vi "SA40144C.20201219 Data Analysis.vi"() -> ()   [LabVIEW 2020]
uses:
  <vilib>/Analysis/baseanly.llb/Mean (DBL).vi
  <userlib>/_OpenG.lib/file/file.llb/Build Path - Traditional__ogtk.vi
  <userlib>/LevyLab/LV to ITX/Data/Data.lvclass
  <userlib>/LevyLab/XY Utilities/xy_utilities.lvlib
  <vilib>/Analysis/NI_AALBase.lvlib
panel:
  in  "Temps to keep (Lifespan)":i32=11
  out "Lifespan vs Temp (hrs)":cluster{i32[], dbl[]}[](graph)
  out "E_a":dbl[](array[numeric])
  out "Arrhenius":T1(graph)
  in  "Temps to keep (Arrhenius fit)":i32=11
  out "G2T vs t":T1(graph)
  out "G4T vs t":T1(graph)
  out "G2T vs t 2D":T1(graph)
  out "G4T vs t  2D":T1(graph)
  in  "Source Voltage":dbl=0.1
  in  "Init Temp":i32=275
  in  "Temp Step":i32=5
  in  "Final Temp":i32=325
  in  "Data File":path=path "G:/My Drive/ansom/Data/PPMS 2/SA40144C.20201219/01 - Temp Sweep/SA40144C.20201219.275K.dat"
  in  "Trimming":i32=400
  in  "Update":bool
  in  "OK":bool
  out "error out":errorcluster
  in  "error in (no error)":errorcluster
  # "2T"
  # "4T"
  # "2T 2D"
  # "4T 2D"
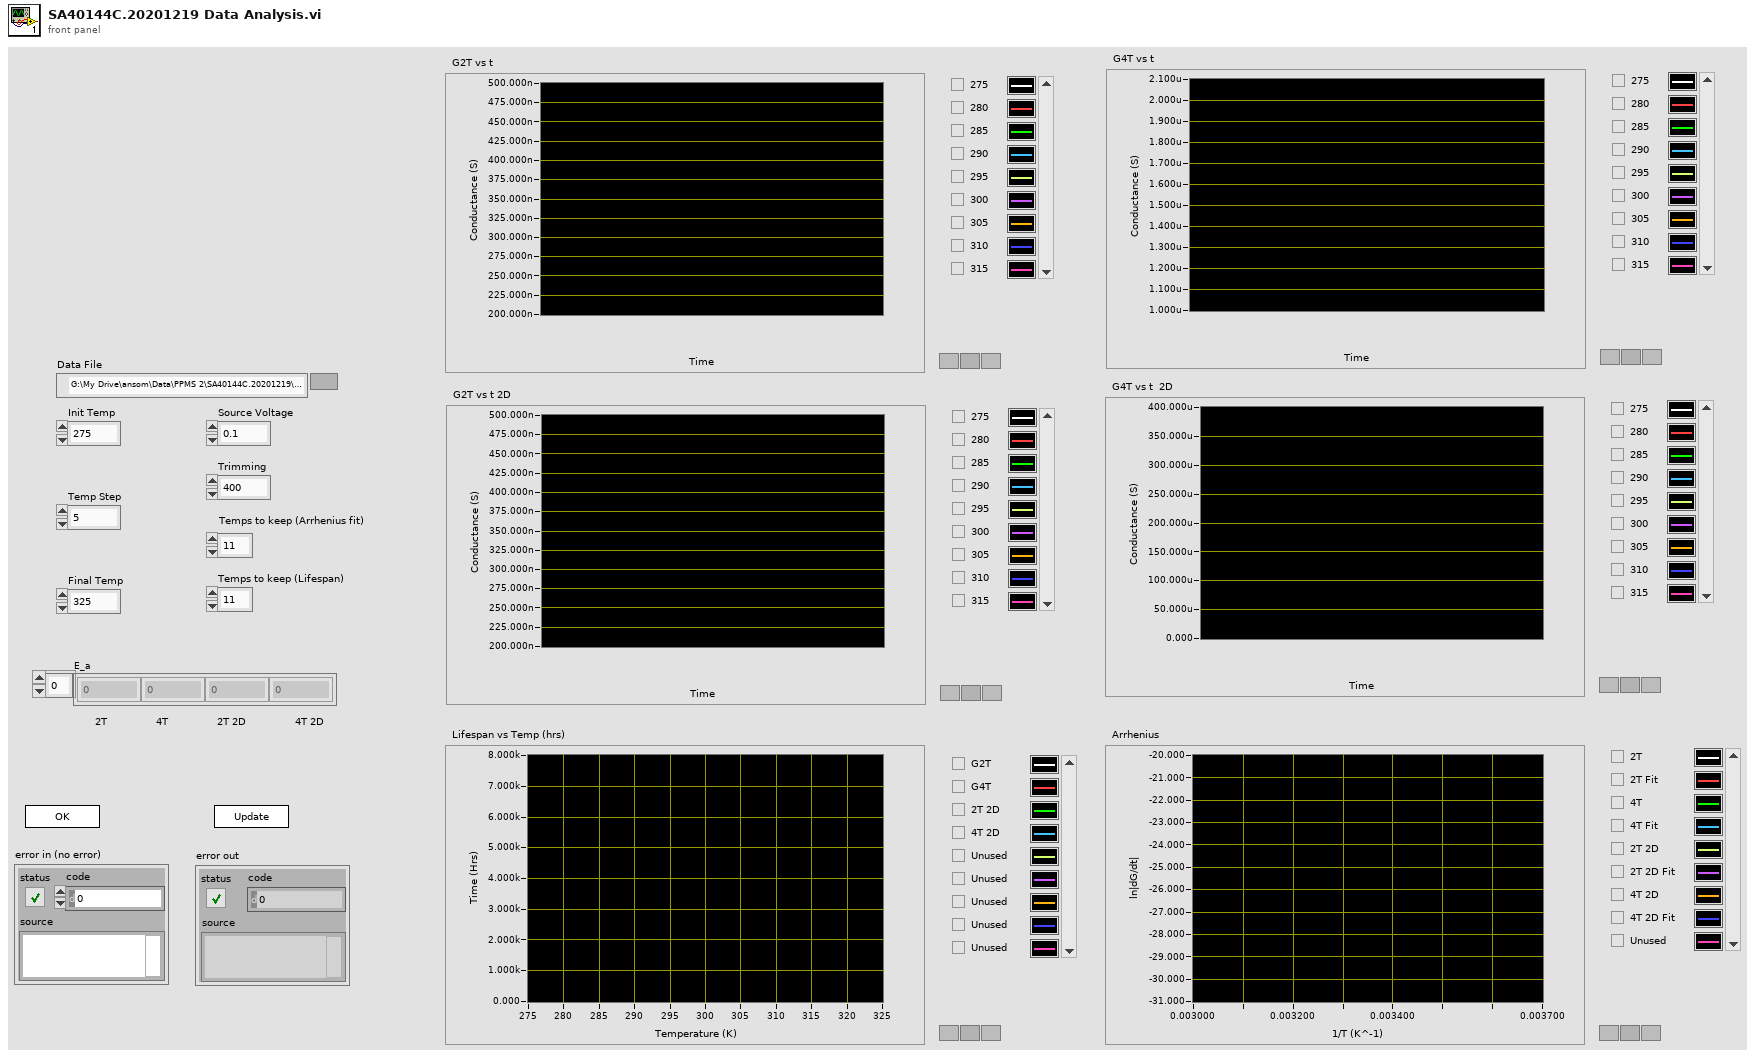
[diagram p1: front panel]
types:
  T1 = cluster{"Data":dbl[], "Best Exponential Fit":dbl[]}[]
  T2 = enum32{"Invalid", "Standard", "Closed", "Hidden", "Minimized", "Maximized"}
  T3 = enum32{"invalid app kind", "Development System", "Run Time System", "Student Edition", "Embedded LabVIEW", "Evaluation", "Custom"}
  T4 = cluster{"Core":cluster{"Current VI Reference":refnum<vi>, "Close Panel on Exit?":bool}, "G2T 1D":cluster{dbl[], dbl[]}[], "G4T 1D":cluster{dbl[], dbl[]}[], "G2T 2D":cluster{dbl[], dbl[]}[], "G4T 2D":cluster{dbl[], dbl[]}[], "Source Voltage":dbl, "Final Temp":i32, "Init Temp":i32, "Temp Step":i32, "Data File":path, "Trimming":i32}
  T5 = cluster{"Current VI Reference":refnum<vi>, "Close Panel on Exit?":bool}
  T6 = typedef "Data.lvclass/Dictionary--cluster.ctl" = cluster{"key":string, "value":variant}
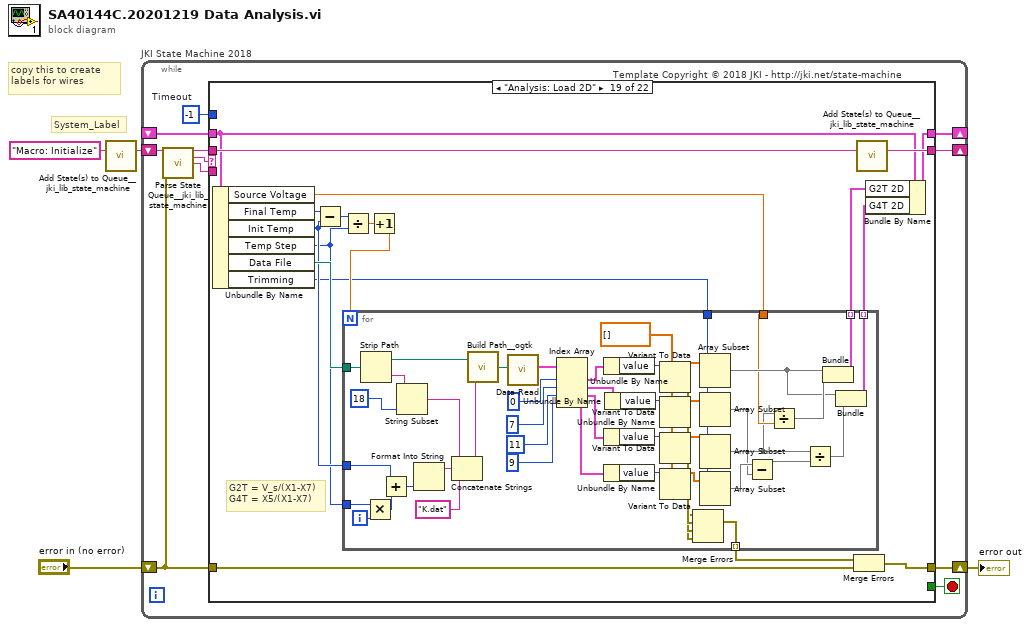
[diagram p0: block diagram]
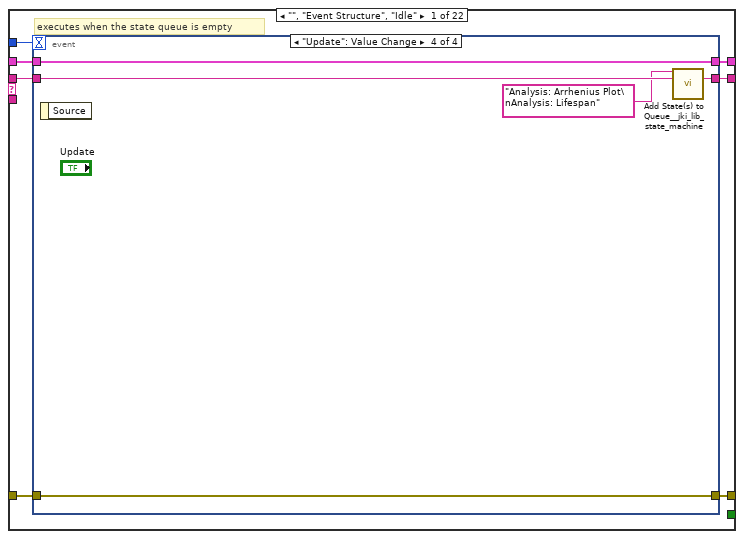
[diagram p2: hidden frame]
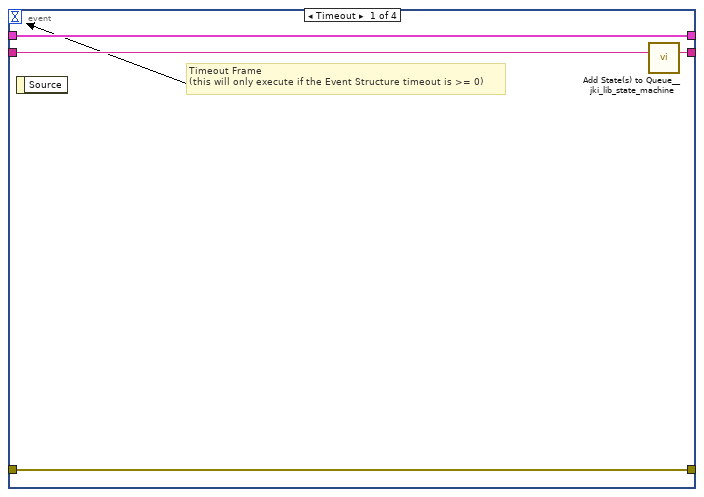
[diagram p3: hidden frame]
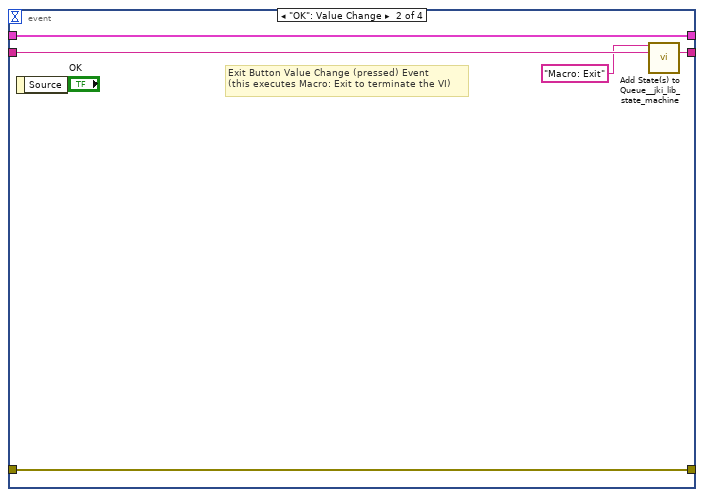
[diagram p4: hidden frame]
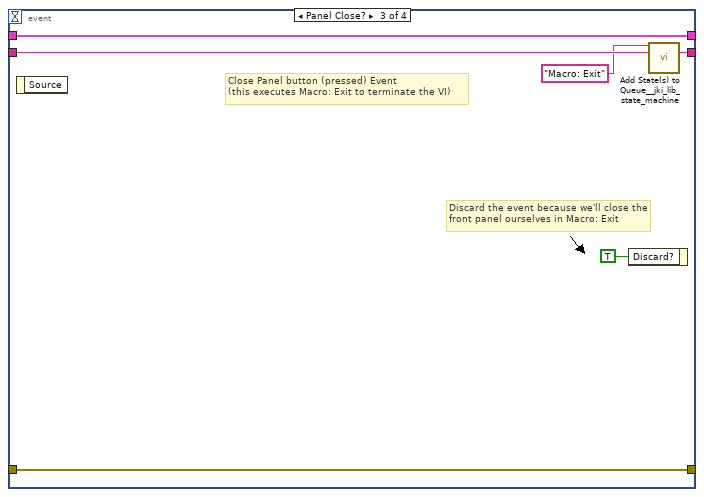
[diagram p5: hidden frame]
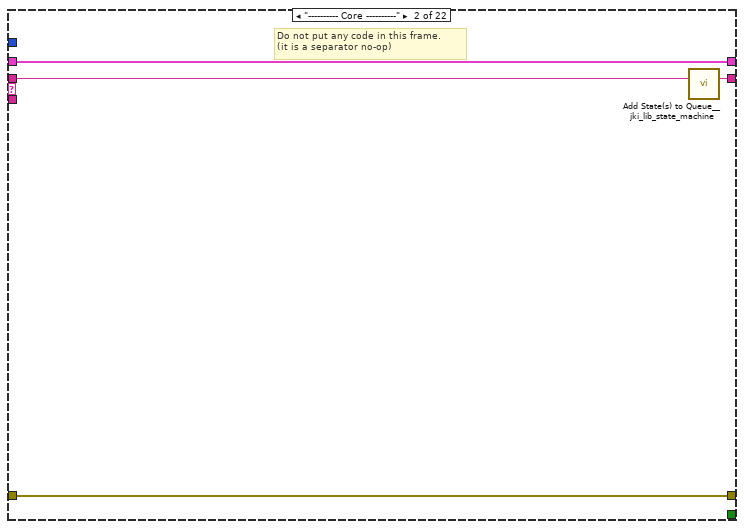
[diagram p6: hidden frame]
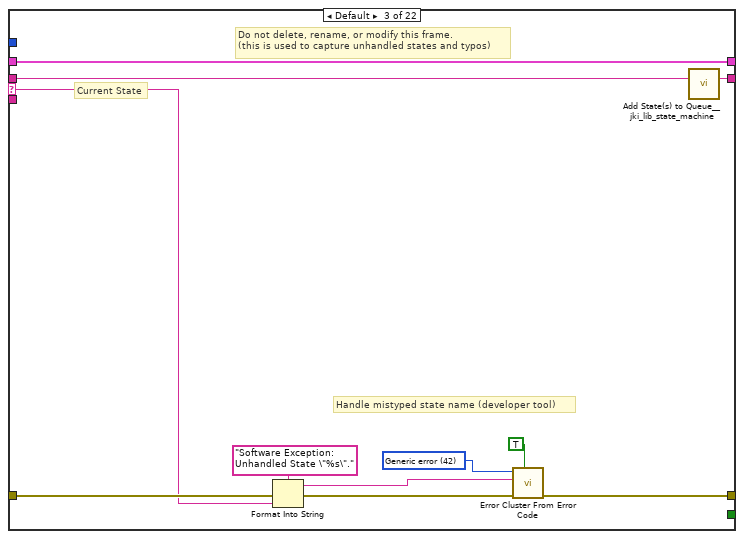
[diagram p7: hidden frame]
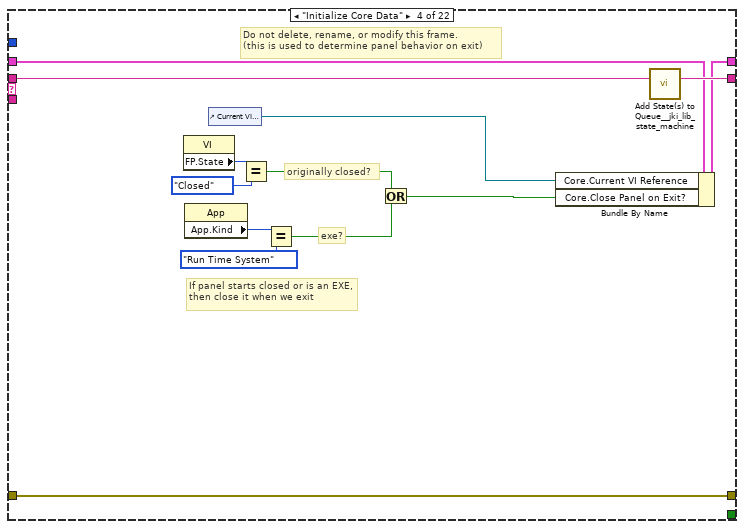
[diagram p8: hidden frame]
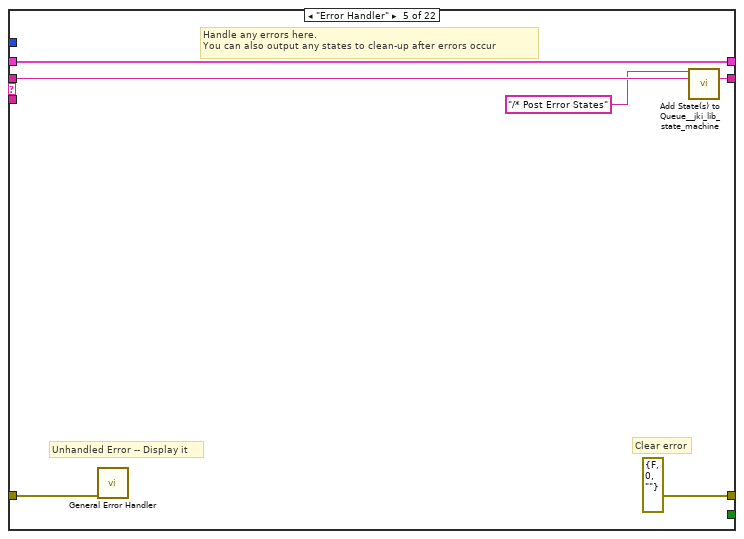
[diagram p9: hidden frame]
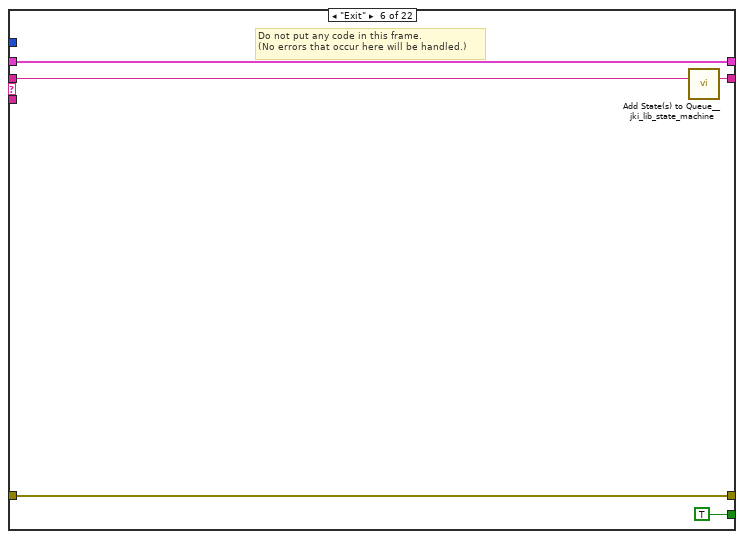
[diagram p10: hidden frame]
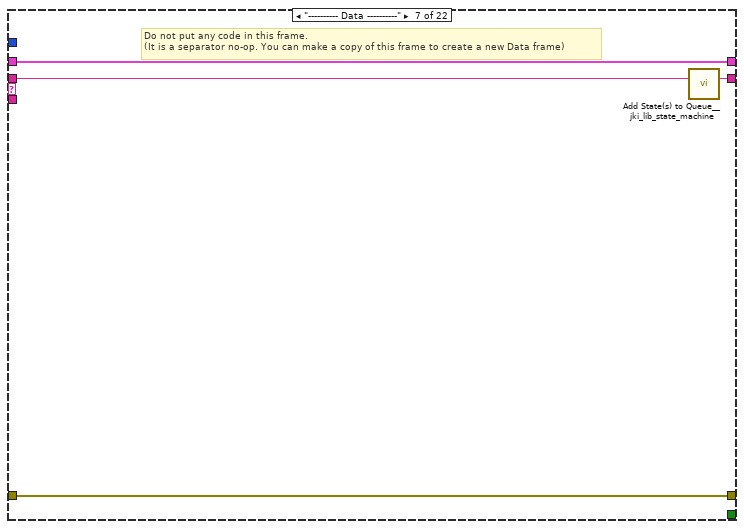
[diagram p11: hidden frame]
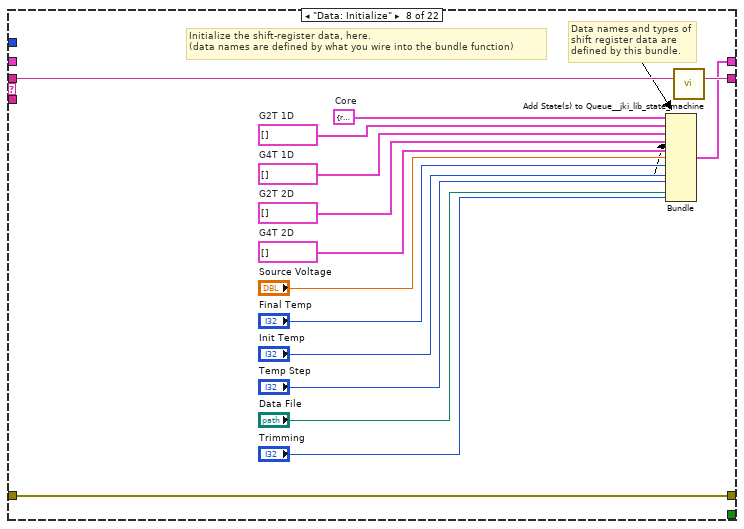
[diagram p12: hidden frame]
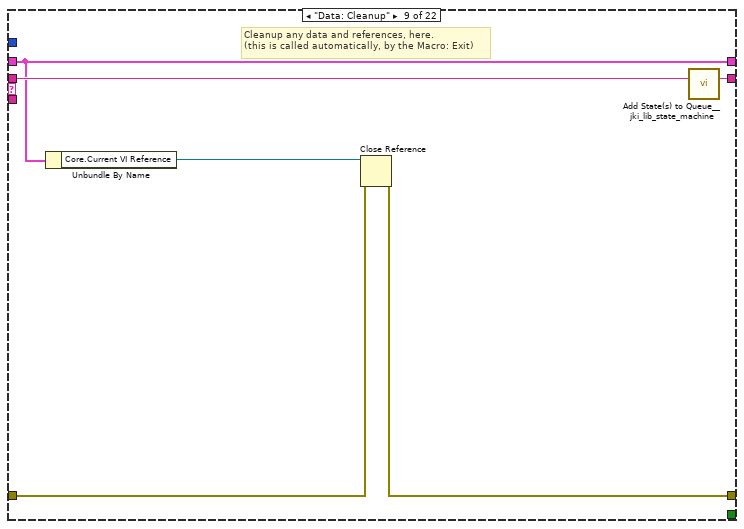
[diagram p13: hidden frame]
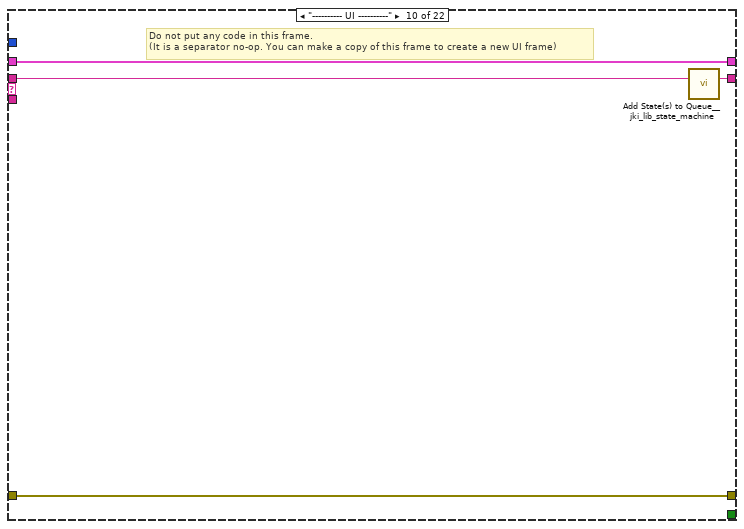
[diagram p14: hidden frame]
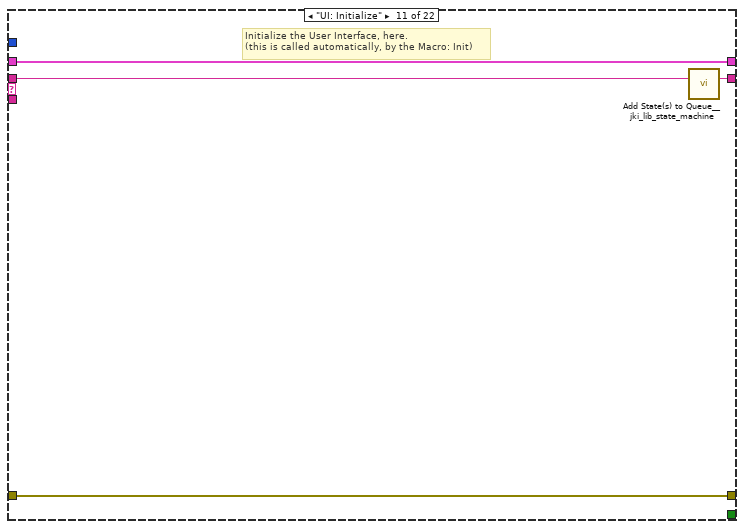
[diagram p15: hidden frame]
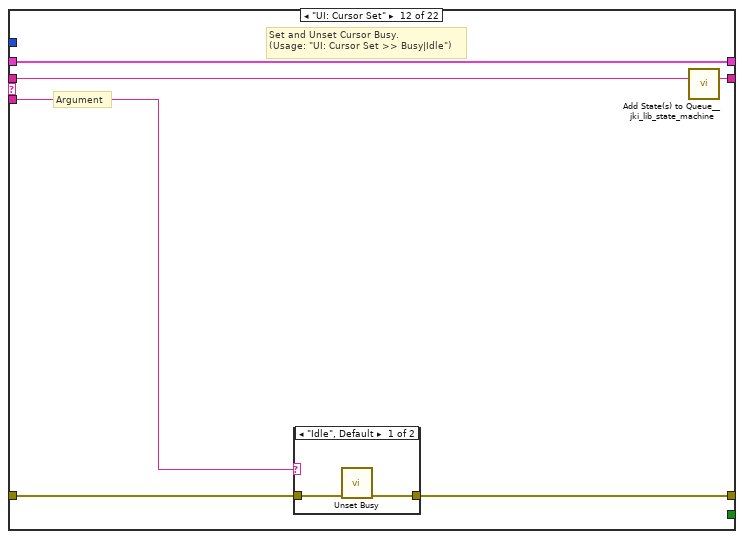
[diagram p16: hidden frame]
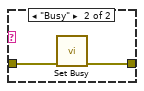
[diagram p17: hidden frame]
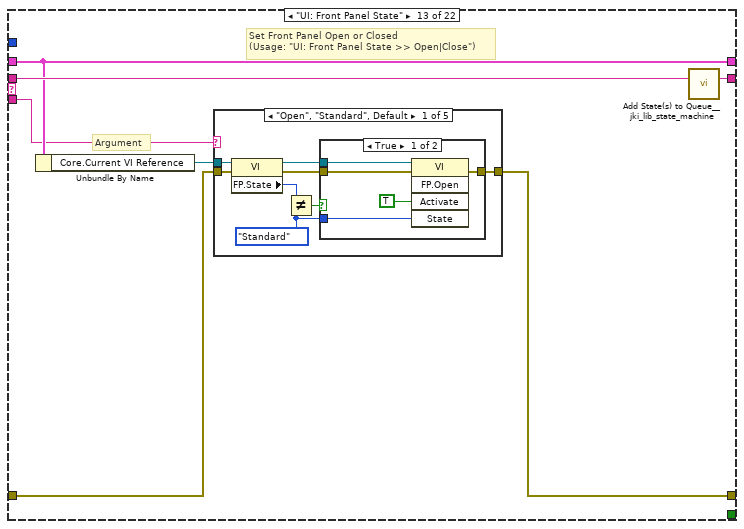
[diagram p18: hidden frame]
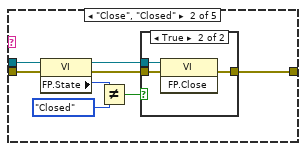
[diagram p20: hidden frame]
diagram:
  # "copy this to create labels for wires"
  # "System_Label"
  n1 = call <vilib>:"Add State(s) to Queue__jki_lib_state_machine.vi"("State(s) in (\"\")"="Macro: Initialize") -> ("States Out"=w4:string)  [unwired: 14 in]
  n2 = while "JKI State Machine 2018" {
    shift-right: [w8] -> _
    shift-left: _ -> [w7]
    shift-right: [w11] -> w1
    shift-left: "error in (no error)" -> [w5]
    shift-right: [w10] -> _
    shift-left: w4 -> [w12]
    stop <- w9 stop-if-true
    w6 = -1  # Timeout
    # "Template Copyright © 2018 JKI - http://jki.net/state-machine"
    n3 = call <vilib>:"Parse State Queue__jki_lib_state_machine.vi"("State Queue"=w12, "Error In (no error)"=w5) -> ("Remaining States"=w14:string, "Current State"=w15:string, "Arguments"=w13:string)  [unwired: 11 in]
    n4 = case shown="\"Analysis: Load 2D\"" w15 {
      selector: w15 -> [_ _ w47 _ _ _ _ _ _ _ _ _ _ _ _ _ _ _ _ _ _ _]
      tunnel: w14 -> [w22 w46 w51 w70 w76 w81 w85 w100 w106 w110 w114 w120 w131 w200 w205 w215 w219 w237 w303 w359 w403 w460]
      tunnel: w13 -> [_ _ _ _ _ _ _ _ _ _ _ w115 w125 _ _ _ _ _ _ _ _ _]
      tunnel: w7 -> [w20 w43 w49 w63 w73 w79 w82 _ w101 w107 w112 w118 w127 w197 w202 w212 w216 w229 w287 w356 w400 w440]
      tunnel: [w19 w44 w53 w67 errorcluster {"status"=FALSE, "code"=0, "source"=""} ("error out") w78 w83 w97 w102 w108 w111 w116 w128 w198 w203 w213 w217 w232 w301 w357 w401 w458] -> w11
      tunnel: w5 -> [w18 w44 w52 w67 w72 w78 w83 w97 w103 w108 w111 w117 w129 w198 w203 w213 w217 w233 w300 w357 w401 w458]
      tunnel: [w21 w45 w50 w69 w75 w80 w84 w99 w105 w109 w113 w119 w130 w199 w204 w214 w218 w236 w302 w358 w402 w459] -> w10
      tunnel: [_ _ _ _ _ TRUE _ _ _ _ _ _ _ _ _ _ _ _ _ _ _ _] -> w9
      tunnel: [w17 w43 w49 w68 w73 w79 w82 w98 w101 w107 w112 w118 w127 w197 w202 w212 w216 w230 w288 w356 w400 w440] -> w8
      tunnel: w6 -> [w16 _ _ _ _ _ _ _ _ _ _ _ _ _ _ _ _ _ _ _ _ _]
      frame "", "Event Structure", "Idle" {
        # "executes when the state queue is empty"
        n5 = event shown="[3] \"Update\": Value Change" {
          selector: _ -> [_ _ _ _]
          dyn-events: _ -> [_ _ _ _]
          timeout: w16 -> [_ _ _ _]
          tunnel: w22 -> [w26 w31 w37 w41]
          tunnel: [w25 w30 w36 w40] -> w21
          tunnel: w20 -> [w23 w28 w34 w42]
          tunnel: [w24 w29 w35 w38] -> w19
          tunnel: w18 -> [w24 w29 w35 w38]
          tunnel: [w23 w28 w34 w42] -> w17
          event Timeout {
            # "Timeout Frame\n(this will only execute if the Event Structure timeout is >= 0)"
            n6 = event-data() -> ()  [unwired: 1 in, 1 out]
            n7 = call <vilib>:"Add State(s) to Queue__jki_lib_state_machine.vi"("State(s) in (\"\")"=w26) -> ("States Out"=w25:string)  [unwired: 14 in]
          }
          event "OK": Value Change {
            # "Exit Button Value Change (pressed) Event\n(this executes Macro: Exit to terminate the VI)"
            n8 = event-data() -> ()  [unwired: 1 in, 1 out]
            n9 = call <vilib>:"Add State(s) to Queue__jki_lib_state_machine.vi"("State(s) in Front (\"\")"="Macro: Exit", "State(s) in (\"\")"=w31) -> ("States Out"=w30:string)  [unwired: 13 in]
          }
          event Panel Close? {
            # "Discard the event because we'll close the front panel ourselves in Macro: Exit"
            # "Close Panel button (pressed) Event\n(this executes Macro: Exit to terminate the VI)"
            n10 = event-data() -> ()  [unwired: 1 in, 1 out]
            n11 = event-data("Discard?"=TRUE) -> ()  [unwired: 1 in, 1 out]
            n12 = call <vilib>:"Add State(s) to Queue__jki_lib_state_machine.vi"("State(s) in Front (\"\")"="Macro: Exit", "State(s) in (\"\")"=w37) -> ("States Out"=w36:string)  [unwired: 13 in]
          }
          event "Update": Value Change {
            n13 = event-data() -> ()  [unwired: 1 in, 1 out]
            n14 = call <vilib>:"Add State(s) to Queue__jki_lib_state_machine.vi"("State(s) in Front (\"\")"="Analysis: Arrhenius Plot\nAnalysis: Lifespan" ("State(s) in Front (\"\")"), "State(s) in (\"\")"=w41) -> ("States Out"=w40:string)  [unwired: 13 in]
          }
        }
      }
      frame "---------- Core ----------" {
        # "Do not put any code in this frame.\n(it is a separator no-op)"
        n15 = call <vilib>:"Add State(s) to Queue__jki_lib_state_machine.vi"("State(s) in (\"\")"=w46) -> ("States Out"=w45:string)  [unwired: 14 in]
      }
      frame Default {
        w56 = 42 items=["No error", "Argument error", "Memory is full", "Out of zone", "End of file", "File already open", "Generic file I/O error", "File not found", "File permission error", "Disk is full", "Duplicate path", "Too many files open", "System feature not enabled", "Resource file not found", "Cannot add resource", "Resource not found", "Image not found", "Image memory error", "Pen does not exist", "Config type invalid", "Config token not found", "Config parse error", "Config memory error", "Bad external code format", "Bad external code offset", "External code not present", "Null window", "Destroy window error", "Null menu", "Print aborted", "Bad print record", "Print driver error", "Windows error during printing", "Memory error during printing", "Print dialog error", "Generic print error", "Invalid device refnum", "Device not found", "Device parameter error", "Device unit error", "Cannot open device", "Device call aborted", "Generic error", "Cancelled by user", "Object ID too low", "Object ID too high", "Object not in heap", "Unknown heap", "Unknown object (invalid DefProc)", "Unknown object (DefProc not in table)", "Message out of range", "Invalid (null) method", "Unknown message", "Manager call not supported", "Bad address", "Network operation in progress", "Network operation timed out", "Connection is busy", "Network attribute not supported", "Network error", "Address in use", "System out of memory", "Connection aborted", "Connection refused", "Not connected", "Already connected", "Connection closed", "Initialization error (interapplication manager)", "Bad occurrence", "Wait on unbound occurrence handler", "Occurrence queue overflow", "Datalog type conflict", "Unused", "Unrecognized type (interapplication manager)", "Memory corrupt", "Failed to make temporary DLL", "Old CIN version", "Drag socket not found", "Failed to load drop-object", "Failed to register OLE object", "Failed to release OLE object", "Format specifier type mismatch", "Unknown format specifier", "Too few format specifiers", "Too many format specifiers", "Scan failed", "Newer CIN version", "Error converting to variant", "Runtime menu error", "Password tampered", "Variant attribute not found", "Incompatible variant data type", "Event data is not available", "Event Store is not present", "Occurrence is not found", "Event Queue is not created", "Event info is not available", "Refnum passed is NULL", "Error retrieving Class GUID", "Error retrieving CoClass GUID", "Error retrieving TypeLib GUID.", "Bad built application magic bytes.", "Specific driver is different from the specific driver associated with the Logical Name.", "There is no session opened to the class driver.", "Max Error", "MAX - Error with config objects", "MAX - Error loading configuration", "MAX - Group not supported"]
        # "Current State"
        # "Do not delete, rename, or modify this frame.\n(this is used to capture unhandled states and typos)"
        # "Handle mistyped state name (developer tool)"
        n16 = Format Into String(format string="Software Exception: Unhandled State \"%s\"." ("message"), error in=w52, w47) -> (resulting string=w55:string, error out=w54:errorcluster)  [unwired: 1 in]
        n17 = call <vilib>:"Error Cluster From Error Code.vi"("show call chain? (False)"=TRUE, "error in (no error)"=w54, "error message (\"\")"=w55, "error code (0)"=w56) -> ("error out"=w53:errorcluster)  [unwired: 5 in]
        n18 = call <vilib>:"Add State(s) to Queue__jki_lib_state_machine.vi"("State(s) in (\"\")"=w51) -> ("States Out"=w50:string)  [unwired: 14 in]
      }
      frame "Initialize Core Data" {
        # "Do not delete, rename, or modify this frame.\n(this is used to determine panel behavior on exit)"
        # "originally closed?"
        # "exe?"
        # "If panel starts closed or is an EXE, then close it when we exit"
        n19 = property class="VI"() -> ("FP.State"=w60:T2)  [unwired: 2 in, 2 out]
        n20 = property class="App"() -> ("App.Kind"=w66:T3)  [unwired: 2 in, 2 out]
        n21 = control-ref of="Current VI Reference"() -> (w61:refnum<vi>)
        n22 = Equal?(x=w60, y=T2."Closed" ("Front Panel Window:State")) -> (x = y?=w58:bool)
        n23 = Equal?(x=w66, y=T3."Run Time System" ("Application:Kind")) -> (x = y?=w64:bool)
        n24 = Or(x=w58, y=w64) -> (x .or. y?=w62:bool)
        n25 = Bundle By Name(cluster=w63, "Core.Current VI Reference"=w61, "Core.Close Panel on Exit?"=w62) -> (w68:T4)
        n26 = call <vilib>:"Add State(s) to Queue__jki_lib_state_machine.vi"("State(s) in (\"\")"=w70) -> ("States Out"=w69:string)  [unwired: 14 in]
      }
      frame "Error Handler" {
        # "Unhandled Error -- Display it"
        # "Handle any errors here.\nYou can also output any states to clean-up after errors occur"
        # "Clear error"
        n27 = call <vilib>:"General Error Handler.vi"("error in (no error)"=w72) -> ()  [unwired: 10 in, 5 out]
        n28 = call <vilib>:"Add State(s) to Queue__jki_lib_state_machine.vi"("State(s) in Front (\"\")"="/* Post Error States", "State(s) in (\"\")"=w76) -> ("States Out"=w75:string)  [unwired: 13 in]
      }
      frame "Exit" {
        # "Do not put any code in this frame.\n(No errors that occur here will be handled.)"
        n29 = call <vilib>:"Add State(s) to Queue__jki_lib_state_machine.vi"("State(s) in (\"\")"=w81) -> ("States Out"=w80:string)  [unwired: 14 in]
      }
      frame "---------- Data ----------" {
        # "Do not put any code in this frame.\n(It is a separator no-op. You can make a copy of this frame to create a new Data frame)"
        n30 = call <vilib>:"Add State(s) to Queue__jki_lib_state_machine.vi"("State(s) in (\"\")"=w85) -> ("States Out"=w84:string)  [unwired: 14 in]
      }
      frame "Data: Initialize" {
        w94 = cluster{dbl[], dbl[]}[] []  # G4T 2D
        w93 = cluster{dbl[], dbl[]}[] []  # G2T 2D
        w92 = cluster{dbl[], dbl[]}[] []  # G4T 1D
        w91 = cluster{dbl[], dbl[]}[] []  # G2T 1D
        w96 = T5 {"Current VI Reference"=refnum, "Close Panel on Exit?"=FALSE}  # Core
        # "Data names and types of shift register data are defined by this bundle."
        # "Initialize the shift-register data, here.\n(data names are defined by what you wire into the bundle function)"
        n31 = Bundle("Core"=w96, "G2T 1D"=w91, "G4T 1D"=w92, "G2T 2D"=w93, "G4T 2D"=w94, "Source Voltage"="Source Voltage", "Final Temp"="Final Temp", "Init Temp"="Init Temp", "Temp Step"="Temp Step", "Data File"="Data File", "Trimming"="Trimming") -> (w98:T4)  [unwired: 1 in]
        n32 = call <vilib>:"Add State(s) to Queue__jki_lib_state_machine.vi"("State(s) in (\"\")"=w100) -> ("States Out"=w99:string)  [unwired: 14 in]
      }
      frame "Data: Cleanup" {
        # "Cleanup any data and references, here.\n(this is called automatically, by the Macro: Exit)"
        n33 = Unbundle By Name(w101) -> ("Core.Current VI Reference"=w104:refnum<vi>)
        n34 = Close Reference(reference=w104, error in (no error)=w103) -> (error out=w102:errorcluster)
        n35 = call <vilib>:"Add State(s) to Queue__jki_lib_state_machine.vi"("State(s) in (\"\")"=w106) -> ("States Out"=w105:string)  [unwired: 14 in]
      }
      frame "---------- UI ----------" {
        # "Do not put any code in this frame.\n(It is a separator no-op. You can make a copy of this frame to create a new UI frame)"
        n36 = call <vilib>:"Add State(s) to Queue__jki_lib_state_machine.vi"("State(s) in (\"\")"=w110) -> ("States Out"=w109:string)  [unwired: 14 in]
      }
      frame "UI: Initialize" {
        # "Initialize the User Interface, here.\n(this is called automatically, by the Macro: Init)"
        n37 = call <vilib>:"Add State(s) to Queue__jki_lib_state_machine.vi"("State(s) in (\"\")"=w114) -> ("States Out"=w113:string)  [unwired: 14 in]
      }
      frame "UI: Cursor Set" {
        # "Argument"
        # "Set and Unset Cursor Busy.\n(Usage: \"UI: Cursor Set >> Busy|Idle\")"
        n38 = case shown="\"Idle\", Default" w115 {
          tunnel: w117 -> [w122 w124]
          tunnel: [w121 w123] -> w116
          frame "Idle", Default {
            n39 = call <vilib>:"Unset Busy.vi"("error in (no error)"=w122) -> ("error out"=w121:errorcluster)  [unwired: 10 in]
          }
          frame "Busy" {
            n40 = call <vilib>:"Set Busy.vi"("error in (no error)"=w124) -> ("error out"=w123:errorcluster)  [unwired: 9 in, 1 out]
          }
        }
        n41 = call <vilib>:"Add State(s) to Queue__jki_lib_state_machine.vi"("State(s) in (\"\")"=w120) -> ("States Out"=w119:string)  [unwired: 14 in]
      }
      frame "UI: Front Panel State" {
        # "Argument"
        # "Set Front Panel Open or Closed\n(Usage: \"UI: Front Panel State >> Open|Close\")"
        n42 = Unbundle By Name(w127) -> ("Core.Current VI Reference"=w126:refnum<vi>)
        n43 = case shown="\"Open\", \"Standard\", Default" w125 {
          tunnel: w129 -> [w137 w152 w163 w176 w189]
          tunnel: [w139 w153 w165 w178 w191] -> w128
          tunnel: w126 -> [w138 w150 w164 w177 w190]
          frame "Open", "Standard", Default {
            w132 = T2."Standard" ("State")
            n44 = property class="VI"(reference=w138, error in=w137) -> (reference out=w135:refnum<vi>, error out=w136:errorcluster, "FP.State"=w134:T2)
            n45 = Not Equal?(x=w134, y=w132) -> (x != y?=w133:bool)
            n46 = case shown="True" w133 {
              tunnel: [w143 w145] -> w139
              tunnel: w136 -> [w142 w145]
              tunnel: w135 -> [w141 _]
              tunnel: w132 -> [w140 _]
              frame True {
                n47 = invoke class="VI" method="FP.Open"(reference=w141, error in=w142, "Activate"=TRUE, "State"=w140) -> (error out=w143:errorcluster)  [unwired: 1 in, 4 out]
              }
              frame False {
              }
            }
          }
          frame "Close", "Closed" {
            n48 = property class="VI"(reference=w150, error in=w152) -> (reference out=w149:refnum<vi>, error out=w151:errorcluster, "FP.State"=w147:T2)
            n49 = Not Equal?(x=w147, y=T2."Closed" ("Front Panel Window:State")) -> (x != y?=w146:bool)
            n50 = case shown="True" w146 {
              tunnel: [w154 w157] -> w153
              tunnel: w151 -> [w154 w156]
              tunnel: w149 -> [_ w155]
              frame False {
              }
              frame True {
                n51 = invoke class="VI" method="FP.Close"(reference=w155, error in=w156) -> (error out=w157:errorcluster)  [unwired: 1 in, 2 out]
              }
            }
          }
          frame "Hidden", "Hide" {
            w158 = T2."Hidden" ("State")
            n52 = property class="VI"(reference=w164, error in=w163) -> (reference out=w161:refnum<vi>, error out=w162:errorcluster, "FP.State"=w160:T2)
            n53 = Not Equal?(x=w160, y=w158) -> (x != y?=w159:bool)
            n54 = case shown="True" w159 {
              tunnel: [w169 w170] -> w165
              tunnel: w162 -> [w168 w170]
              tunnel: w161 -> [w167 _]
              tunnel: w158 -> [w166 _]
              frame True {
                n55 = invoke class="VI" method="FP.Open"(reference=w167, error in=w168, "State"=w166) -> (error out=w169:errorcluster)  [unwired: 2 in, 4 out]
              }
              frame False {
              }
            }
          }
          frame "Minimize", "Minimized" {
            w171 = T2."Minimized" ("State")
            n56 = property class="VI"(reference=w177, error in=w176) -> (reference out=w174:refnum<vi>, error out=w175:errorcluster, "FP.State"=w173:T2)
            n57 = Not Equal?(x=w173, y=w171) -> (x != y?=w172:bool)
            n58 = case shown="True" w172 {
              tunnel: [w182 w183] -> w178
              tunnel: w175 -> [w181 w183]
              tunnel: w174 -> [w180 _]
              tunnel: w171 -> [w179 _]
              frame True {
                n59 = invoke class="VI" method="FP.Open"(reference=w180, error in=w181, "State"=w179) -> (error out=w182:errorcluster)  [unwired: 2 in, 4 out]
              }
              frame False {
              }
            }
          }
          frame "Maximize", "Maximized" {
            w184 = T2."Maximized" ("State")
            n60 = property class="VI"(reference=w190, error in=w189) -> (reference out=w187:refnum<vi>, error out=w188:errorcluster, "FP.State"=w186:T2)
            n61 = Not Equal?(x=w186, y=w184) -> (x != y?=w185:bool)
            n62 = case shown="True" w185 {
              tunnel: [w195 w196] -> w191
              tunnel: w188 -> [w194 w196]
              tunnel: w187 -> [w193 _]
              tunnel: w184 -> [w192 _]
              frame True {
                n63 = invoke class="VI" method="FP.Open"(reference=w193, error in=w194, "State"=w192) -> (error out=w195:errorcluster)  [unwired: 2 in, 4 out]
              }
              frame False {
              }
            }
          }
        }
        n64 = call <vilib>:"Add State(s) to Queue__jki_lib_state_machine.vi"("State(s) in (\"\")"=w131) -> ("States Out"=w130:string)  [unwired: 14 in]
      }
      frame "---------- Macro ----------" {
        # "Do not put any code in this frame.\n(It is a separator no-op. You can make a copy of this frame to create a new Macro frame)"
        n65 = call <vilib>:"Add State(s) to Queue__jki_lib_state_machine.vi"("State(s) in (\"\")"=w200) -> ("States Out"=w199:string)  [unwired: 14 in]
      }
      frame "Macro: Initialize" {
        # "Initialization Macro\n(This is called once, when the VI starts)"
        n66 = call <vilib>:"Add State(s) to Queue__jki_lib_state_machine.vi"("State(s) in Front (\"\")"="Data: Initialize\nInitialize Core Data\nUI: Initialize\nUI: Front Panel State >> Open\nAnalysis: Load 1D\nAnalysis: Load 2D\nAnalysis: Plot G vs t\nAnalysis: Arrhenius Plot\nAnalysis: Lifespan", "State(s) in (\"\")"=w205) -> ("States Out"=w204:string)  [unwired: 13 in]
      }
      frame "Macro: Exit" {
        # "Exit Macro\n(This is called once, when the VI exits)"
        n67 = Unbundle By Name(w212) -> ("Core.Close Panel on Exit?"=w211:bool)
        n68 = Select(t="UI: Front Panel State >> Close", s=w211, f="") -> (s? t:f=w208:string)
        n69 = call <vilib>:"Add State(s) to Queue__jki_lib_state_machine.vi"("State(s) in (\"\")"=w208, "State(s) at Back (\"\")"="Data: Cleanup\nExit") -> ("States Out"=w206:string)  [unwired: 13 in]
        n70 = call <vilib>:"Add State(s) to Queue__jki_lib_state_machine.vi"("State(s) in Front (\"\")"=w206, "State(s) in (\"\")"=w215) -> ("States Out"=w214:string)  [unwired: 13 in]
      }
      frame "---------- Analysis ----------" {
        # "Template Separator\n(You can make a copy of, or modify, this frame)"
        n71 = call <vilib>:"Add State(s) to Queue__jki_lib_state_machine.vi"("State(s) in (\"\")"=w219) -> ("States Out"=w218:string)  [unwired: 14 in]
      }
      frame "Analysis: Load 1D" {
        # "G2T = V_s/(X1-X7)\nG4T = X5/(X1-X7)"
        n72 = Unbundle By Name(w229) -> ("Source Voltage"=w228:dbl, "Final Temp"=w225:i32, "Init Temp"=w222:i32, "Temp Step"=w221:i32, "Data File"=w223:path, "Trimming"=w220:i32)
        n73 = Subtract(x=w225, y=w222) -> (x-y=w234:i32)
        n74 = Divide(x=w234, y=w221) -> (x/y=w235:dbl)
        n75 = Increment(x=w235) -> (x+1=w224:dbl)
        n76 = for {
          N: w224 -> [_]
          tunnel: [w257] -> w231 mode=indexing
          tunnel: w228 -> [w238]
          tunnel: [w252] -> w227 mode=indexing
          tunnel: [w251] -> w226 mode=indexing
          tunnel: w223 -> [w250]
          tunnel: w222 -> [w249]
          tunnel: w221 -> [w248]
          tunnel: w220 -> [w247]
          i -> [w276]
          w267 = dbl[] []
          n77 = Strip Path(path=w250) -> (stripped path=w281:path, name=w280:string)
          n78 = Multiply(x=w248, y=w276) -> (x*y=w277:i32)
          n79 = Add(x=w249, y=w277) -> (x+y=w282:i32)
          n80 = String Subset(string=w280, length (rest)=18) -> (substring=w278:string)  [unwired: 1 in]
          n81 = Format Into String(w282) -> (resulting string=w284:string)  [unwired: 3 in, 1 out]
          n82 = Concatenate Strings(w278, w284, "K.dat" ("string")) -> (w283:string)
          n83 = call-poly <userlib>:"Build Path__ogtk.vi"("name or relative path"=w283, "base path"=w281) -> ("appended path"=w285:path)
          n84 = call <userlib>:"Data Read.vi"("path"=w285) -> ("Data (Dictionary)"=w270:T6[])  [unwired: 7 in, 3 out]
          n85 = Index Array(array=w270, index #1=0, index #2=3, index #3=11 ("index"), index #4=15) -> (element #1=w262:T6, element #2=w261:T6, element #3=w260:T6, element #4=w259:T6)
          n86 = Unbundle By Name(w262) -> ("value"=w266:variant)
          n87 = Unbundle By Name(w260) -> ("value"=w264:variant)
          n88 = Unbundle By Name(w259) -> ("value"=w263:variant)
          n89 = Unbundle By Name(w261) -> ("value"=w265:variant)
          n90 = Variant To Data(type=w267, Variant=w266) -> (data=w243:dbl[], error out=w258:errorcluster)  [unwired: 1 in]
          n91 = Variant To Data(type=w267, Variant=w265) -> (data=w241:dbl[], error out=w273:errorcluster)  [unwired: 1 in]
          n92 = Variant To Data(type=w267, Variant=w264) -> (data=w244:dbl[], error out=w272:errorcluster)  [unwired: 1 in]
          n93 = Variant To Data(type=w267, Variant=w263) -> (data=w246:dbl[], error out=w271:errorcluster)  [unwired: 1 in]
          n94 = Merge Errors(w258, w273, w272, w271) -> (w257:errorcluster)
          n95 = Array Subset(array=w243, index=w247) -> (w242:dbl[])  [unwired: 1 in]
          n96 = Array Subset(array=w241, index=w247) -> (w240:dbl[])  [unwired: 1 in]
          n97 = Array Subset(array=w244, index=w247) -> (w239:dbl[])  [unwired: 1 in]
          n98 = Array Subset(array=w246, index=w247) -> (w245:dbl[])  [unwired: 1 in]
          n99 = Subtract(x=w245, y=w240) -> (x-y=w256:dbl[])
          n100 = Divide(x=w239, y=w238) -> (x/y=w254:dbl[])
          n101 = Divide(x=w239, y=w256) -> (x/y=w255:dbl[])
          n102 = Bundle(w242, w254) -> (w252:cluster{dbl[], dbl[]})  [unwired: 1 in]
          n103 = Bundle(w242, w255) -> (w251:cluster{dbl[], dbl[]})  [unwired: 1 in]
        }
        n104 = Merge Errors(w231, w233) -> (w232:errorcluster)
        n105 = call <vilib>:"Add State(s) to Queue__jki_lib_state_machine.vi"("State(s) in (\"\")"=w237) -> ("States Out"=w236:string)  [unwired: 14 in]
        n106 = Bundle By Name(cluster=w229, "G2T 1D"=w227, "G4T 1D"=w226) -> (w230:T4)
      }
      frame "Analysis: Load 2D" {
        # "G2T = V_s/(X1-X7)\nG4T = X5/(X1-X7)"
        n107 = Unbundle By Name(w287) -> ("Source Voltage"=w297:dbl, "Final Temp"=w294:i32, "Init Temp"=w291:i32, "Temp Step"=w290:i32, "Data File"=w292:path, "Trimming"=w289:i32)
        n108 = Subtract(x=w294, y=w291) -> (x-y=w298:i32)
        n109 = Divide(x=w298, y=w290) -> (x/y=w299:dbl)
        n110 = Increment(x=w299) -> (x+1=w293:dbl)
        n111 = for {
          N: w293 -> [_]
          tunnel: [w323] -> w286 mode=indexing
          tunnel: w297 -> [w305]
          tunnel: [w318] -> w296 mode=indexing
          tunnel: [w317] -> w295 mode=indexing
          tunnel: w292 -> [w316]
          tunnel: w291 -> [w315]
          tunnel: w290 -> [w314]
          tunnel: w289 -> [w313]
          i -> [w342]
          w333 = dbl[] []
          n112 = Strip Path(path=w316) -> (stripped path=w347:path, name=w346:string)
          n113 = Multiply(x=w314, y=w342) -> (x*y=w343:i32)
          n114 = Add(x=w315, y=w343) -> (x+y=w348:i32)
          n115 = String Subset(string=w346, length (rest)=18) -> (substring=w344:string)  [unwired: 1 in]
          n116 = Format Into String(w348) -> (resulting string=w350:string)  [unwired: 3 in, 1 out]
          n117 = Concatenate Strings(w344, w350, "K.dat" ("string")) -> (w349:string)
          n118 = call-poly <userlib>:"Build Path__ogtk.vi"("name or relative path"=w349, "base path"=w347) -> ("appended path"=w351:path)
          n119 = call <userlib>:"Data Read.vi"("path"=w351) -> ("Data (Dictionary)"=w336:T6[])  [unwired: 7 in, 3 out]
          n120 = Index Array(array=w336, index #1=0, index #2=7, index #3=11 ("index"), index #4=9) -> (element #1=w328:T6, element #2=w327:T6, element #3=w326:T6, element #4=w325:T6)
          n121 = Unbundle By Name(w328) -> ("value"=w332:variant)
          n122 = Unbundle By Name(w326) -> ("value"=w330:variant)
          n123 = Unbundle By Name(w325) -> ("value"=w329:variant)
          n124 = Unbundle By Name(w327) -> ("value"=w331:variant)
          n125 = Variant To Data(type=w333, Variant=w332) -> (data=w309:dbl[], error out=w324:errorcluster)  [unwired: 1 in]
          n126 = Variant To Data(type=w333, Variant=w331) -> (data=w307:dbl[], error out=w339:errorcluster)  [unwired: 1 in]
          n127 = Variant To Data(type=w333, Variant=w330) -> (data=w310:dbl[], error out=w338:errorcluster)  [unwired: 1 in]
          n128 = Variant To Data(type=w333, Variant=w329) -> (data=w312:dbl[], error out=w337:errorcluster)  [unwired: 1 in]
          n129 = Merge Errors(w324, w339, w338, w337) -> (w323:errorcluster)
          n130 = Array Subset(array=w309, index=w313) -> (w308:dbl[])  [unwired: 1 in]
          n131 = Array Subset(array=w307, index=w313) -> (w306:dbl[])  [unwired: 1 in]
          n132 = Array Subset(array=w310, index=w313) -> (w304:dbl[])  [unwired: 1 in]
          n133 = Array Subset(array=w312, index=w313) -> (w311:dbl[])  [unwired: 1 in]
          n134 = Subtract(x=w311, y=w306) -> (x-y=w322:dbl[])
          n135 = Divide(x=w304, y=w305) -> (x/y=w320:dbl[])
          n136 = Divide(x=w304, y=w322) -> (x/y=w321:dbl[])
          n137 = Bundle(w308, w320) -> (w318:cluster{dbl[], dbl[]})  [unwired: 1 in]
          n138 = Bundle(w308, w321) -> (w317:cluster{dbl[], dbl[]})  [unwired: 1 in]
        }
        n139 = Merge Errors(w286, w300) -> (w301:errorcluster)
        n140 = call <vilib>:"Add State(s) to Queue__jki_lib_state_machine.vi"("State(s) in (\"\")"=w303) -> ("States Out"=w302:string)  [unwired: 14 in]
        n141 = Bundle By Name(cluster=w287, "G2T 2D"=w296, "G4T 2D"=w295) -> (w288:T4)
      }
      frame "Analysis: Plot G vs t" {
        n142 = Unbundle By Name(w356) -> ("G2T 1D"=→"G2T vs t":cluster{dbl[], dbl[]}[], "G4T 1D"=→"G4T vs t":cluster{dbl[], dbl[]}[], "G2T 2D"=→"G2T vs t 2D":cluster{dbl[], dbl[]}[], "G4T 2D"=→"G4T vs t  2D":cluster{dbl[], dbl[]}[])
        n143 = call <vilib>:"Add State(s) to Queue__jki_lib_state_machine.vi"("State(s) in (\"\")"=w359) -> ("States Out"=w358:string)  [unwired: 14 in]
      }
      frame "Analysis: Arrhenius Plot" {
        n144 = Unbundle By Name(w400) -> ("G2T 1D"=w363:cluster{dbl[], dbl[]}[], "G4T 1D"=w362:cluster{dbl[], dbl[]}[], "G2T 2D"=w369:cluster{dbl[], dbl[]}[], "G4T 2D"=w371:cluster{dbl[], dbl[]}[], "Final Temp"=w397:i32, "Init Temp"=w395:i32, "Temp Step"=w394:i32)  [unwired: 1 out]
        n145 = Subtract(x=w397, y=w395) -> (x-y=w398:i32)
        n146 = Divide(x=w398, y=w394) -> (x/y=w399:dbl)
        n147 = Increment(x=w399) -> (x+1=w396:dbl)
        n148 = for {
          N: w396 -> [_]
          tunnel: w395 -> [w406]
          tunnel: w394 -> [w407]
          tunnel: [w404] -> w380 mode=indexing
          i -> [w408]
          n149 = Multiply(x=w407, y=w408) -> (x*y=w409:i32)
          n150 = Add(x=w406, y=w409) -> (x+y=w405:i32)
          n151 = Reciprocal(x=w405) -> (1/x=w404:dbl)
        }
        n152 = call-poly <userlib>:"Linear Fit.vi"("XY-data"=w363) -> ("slopes"=w360:dbl[])  [unwired: 4 in, 6 out]
        n153 = call-poly <userlib>:"Linear Fit.vi"("XY-data"=w362) -> ("slopes"=w361:dbl[])  [unwired: 4 in, 6 out]
        n154 = call-poly <userlib>:"Linear Fit.vi"("XY-data"=w369) -> ("slopes"=w368:dbl[])  [unwired: 4 in, 6 out]
        n155 = call-poly <userlib>:"Linear Fit.vi"("XY-data"=w371) -> ("slopes"=w370:dbl[])  [unwired: 4 in, 6 out]
        n156 = Absolute Value(x=w360) -> (abs(x)=w390:dbl[])
        n157 = Absolute Value(x=w361) -> (abs(x)=w391:dbl[])
        n158 = Absolute Value(x=w368) -> (abs(x)=w392:dbl[])
        n159 = Absolute Value(x=w370) -> (abs(x)=w393:dbl[])
        n160 = Natural Logarithm(1:w390) -> (0:w384:dbl[])
        n161 = Natural Logarithm(1:w391) -> (0:w383:dbl[])
        n162 = Natural Logarithm(1:w392) -> (0:w382:dbl[])
        n163 = Natural Logarithm(1:w393) -> (0:w381:dbl[])
        n164 = Array Subset(array=w384, length="Temps to keep (Arrhenius fit)") -> (w378:dbl[])  [unwired: 1 in]
        n165 = Array Subset(array=w383, length="Temps to keep (Arrhenius fit)") -> (w377:dbl[])  [unwired: 1 in]
        n166 = Array Subset(array=w382, length="Temps to keep (Arrhenius fit)") -> (w376:dbl[])  [unwired: 1 in]
        n167 = Array Subset(array=w381, length="Temps to keep (Arrhenius fit)") -> (w375:dbl[])  [unwired: 1 in]
        n168 = Array Subset(array=w380, length="Temps to keep (Arrhenius fit)") -> (w374:dbl[])  [unwired: 1 in]
        n169 = Bundle(w374, w378) -> (w387:cluster{dbl[], dbl[]})  [unwired: 1 in]
        n170 = Bundle(w374, w377) -> (w389:cluster{dbl[], dbl[]})  [unwired: 1 in]
        n171 = Bundle(w374, w376) -> (w388:cluster{dbl[], dbl[]})  [unwired: 1 in]
        n172 = Bundle(w374, w375) -> (w386:cluster{dbl[], dbl[]})  [unwired: 1 in]
        n173 = Build Array(w387, w389, w388, w386) -> (w367:cluster{dbl[], dbl[]}[])
        n174 = call-poly <userlib>:"Linear Fit.vi"("XY-data"=w367) -> ("Best Fits"=w366:cluster{"X-array":dbl[], "Y-array":dbl[]}[], "XY-data out"=w365:cluster{"X-array":dbl[], "Y-array":dbl[]}[], "slopes"=w364:dbl[])  [unwired: 4 in, 4 out]
        n175 = Multiply(x=w364, y=8.617333e-05) -> (x*y=→"E_a":dbl[])
        n176 = Interleave 1D Arrays(w365, w366) -> (→"Arrhenius":cluster{"X-array":dbl[], "Y-array":dbl[]}[])
        n177 = call <vilib>:"Add State(s) to Queue__jki_lib_state_machine.vi"("State(s) in (\"\")"=w403) -> ("States Out"=w402:string)  [unwired: 14 in]
      }
      frame "Analysis: Lifespan" {
        w418 = 3600
        # "Template Separator\n(You can make a copy of, or modify, this frame)"
        n178 = Unbundle By Name(w440) -> ("G2T 1D"=w457:cluster{dbl[], dbl[]}[], "G4T 1D"=w456:cluster{dbl[], dbl[]}[], "G2T 2D"=w455:cluster{dbl[], dbl[]}[], "G4T 2D"=w454:cluster{dbl[], dbl[]}[], "Final Temp"=w451:i32, "Init Temp"=w439:i32, "Temp Step"=w438:i32)  [unwired: 1 out]
        n179 = Subtract(x=w451, y=w439) -> (x-y=w452:i32)
        n180 = Divide(x=w452, y=w438) -> (x/y=w453:dbl)
        n181 = Increment(x=w453) -> (x+1=w437:dbl)
        n182 = for {
          N: w437 -> [_]
          tunnel: w439 -> [w475]
          tunnel: w438 -> [w474]
          tunnel: [w473] -> w436 mode=indexing
          i -> [w476]
          n183 = Multiply(x=w474, y=w476) -> (x*y=w477:i32)
          n184 = Add(x=w475, y=w477) -> (x+y=w473:i32)
        }
        n185 = call <userlib>:"Linear Fit (multiple).vi"("XY-data"=w457) -> ("XY-data out"=w431:cluster{"X-array":dbl[], "Y-array":dbl[]}[], "slopes"=w434:dbl[])  [unwired: 4 in, 5 out]
        n186 = call <userlib>:"Linear Fit (multiple).vi"("XY-data"=w456) -> ("XY-data out"=w430:cluster{"X-array":dbl[], "Y-array":dbl[]}[], "slopes"=w433:dbl[])  [unwired: 4 in, 5 out]
        n187 = call <userlib>:"Linear Fit (multiple).vi"("XY-data"=w455) -> ("XY-data out"=w429:cluster{"X-array":dbl[], "Y-array":dbl[]}[], "slopes"=w432:dbl[])  [unwired: 4 in, 5 out]
        n188 = call <userlib>:"Linear Fit (multiple).vi"("XY-data"=w454) -> ("XY-data out"=w428:cluster{"X-array":dbl[], "Y-array":dbl[]}[], "slopes"=w435:dbl[])  [unwired: 4 in, 5 out]
        n189 = for {
          tunnel: w431 -> [w469] mode=indexing
          tunnel: w430 -> [w470] mode=indexing
          tunnel: w429 -> [w471] mode=indexing
          tunnel: w428 -> [w472] mode=indexing
          tunnel: [w464] -> w427 mode=indexing
          tunnel: [w463] -> w426 mode=indexing
          tunnel: [w462] -> w425 mode=indexing
          tunnel: [w461] -> w424 mode=indexing
          n190 = Unbundle(w469) -> ("Y-array"=w465:dbl[])  [unwired: 1 out]
          n191 = Unbundle(w470) -> ("Y-array"=w466:dbl[])  [unwired: 1 out]
          n192 = Unbundle(w471) -> ("Y-array"=w467:dbl[])  [unwired: 1 out]
          n193 = Unbundle(w472) -> ("Y-array"=w468:dbl[])  [unwired: 1 out]
          n194 = call-poly <vilib>:"Mean.vi"("X"=w468) -> ("mean"=w461:dbl)  [unwired: 1 out]
          n195 = call-poly <vilib>:"Mean.vi"("X"=w467) -> ("mean"=w462:dbl)  [unwired: 1 out]
          n196 = call-poly <vilib>:"Mean.vi"("X"=w466) -> ("mean"=w463:dbl)  [unwired: 1 out]
          n197 = call-poly <vilib>:"Mean.vi"("X"=w465) -> ("mean"=w464:dbl)  [unwired: 1 out]
        }
        n198 = Divide(x=w427, y=w434) -> (x/y=w422:dbl[])
        n199 = Divide(x=w426, y=w433) -> (x/y=w421:dbl[])
        n200 = Divide(x=w425, y=w432) -> (x/y=w420:dbl[])
        n201 = Divide(x=w424, y=w435) -> (x/y=w419:dbl[])
        n202 = Divide(x=w422, y=w418) -> (x/y=w414:dbl[])
        n203 = Divide(x=w421, y=w418) -> (x/y=w415:dbl[])
        n204 = Divide(x=w420, y=w418) -> (x/y=w416:dbl[])
        n205 = Divide(x=w419, y=w418) -> (x/y=w417:dbl[])
        n206 = Array Subset(array=w414, length="Temps to keep (Lifespan)") -> (w445:dbl[])  [unwired: 1 in]
        n207 = Array Subset(array=w415, length="Temps to keep (Lifespan)") -> (w444:dbl[])  [unwired: 1 in]
        n208 = Array Subset(array=w416, length="Temps to keep (Lifespan)") -> (w443:dbl[])  [unwired: 1 in]
        n209 = Array Subset(array=w417, length="Temps to keep (Lifespan)") -> (w442:dbl[])  [unwired: 1 in]
        n210 = Array Subset(array=w436, length="Temps to keep (Lifespan)") -> (w441:i32[])  [unwired: 1 in]
        n211 = Absolute Value(x=w445) -> (abs(x)=w410:dbl[])
        n212 = Absolute Value(x=w444) -> (abs(x)=w411:dbl[])
        n213 = Absolute Value(x=w443) -> (abs(x)=w412:dbl[])
        n214 = Absolute Value(x=w442) -> (abs(x)=w413:dbl[])
        n215 = Bundle(w441, w410) -> (w448:cluster{i32[], dbl[]})  [unwired: 1 in]
        n216 = Bundle(w441, w411) -> (w450:cluster{i32[], dbl[]})  [unwired: 1 in]
        n217 = Bundle(w441, w412) -> (w449:cluster{i32[], dbl[]})  [unwired: 1 in]
        n218 = Bundle(w441, w413) -> (w447:cluster{i32[], dbl[]})  [unwired: 1 in]
        n219 = Build Array(w448, w450, w449, w447) -> (→"Lifespan vs Temp (hrs)":cluster{i32[], dbl[]}[])
        n220 = call <vilib>:"Add State(s) to Queue__jki_lib_state_machine.vi"("State(s) in (\"\")"=w460) -> ("States Out"=w459:string)  [unwired: 14 in]
      }
    }
  }
  "error out" <- w1
